vi "Open.vi"(8 "error in (no error)":errorcluster, 11 "Theory in":refnum<class "Theory.lvclass">) -> (0 "error out":errorcluster, 3 "Theory out":refnum<class "Theory.lvclass">)   [LabVIEW 2017, in "Theory.lvclass"]
doc: "Opens the test."
uses:
  Theory.lvclass
  Theory.lvclass/Theory.ctl
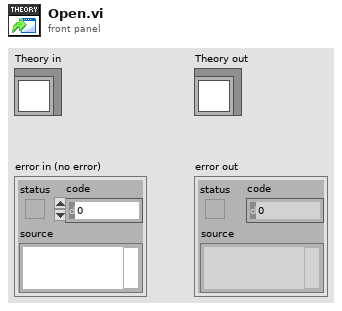
[diagram p1: front panel]
types:
  T1 = enum32{"Invalid", "Standard", "Closed", "Hidden", "Minimized", "Maximized"}
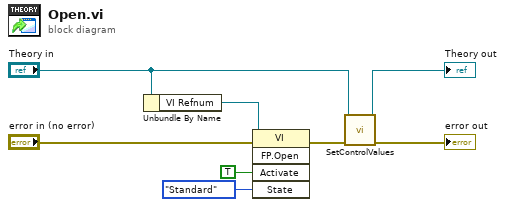
[diagram p0: block diagram]
diagram:
  n1 = Unbundle By Name("Theory in") -> ("VI Refnum"=w8:refnum<vi>)
  n2 = invoke class="VI" method="FP.Open"(reference=w8, error in="error in (no error)", "Activate"=TRUE ("Activate?"), "State"=T1."Standard") -> (error out=w4:errorcluster)  [unwired: 1 in, 4 out]
  n3 = call "SetControlValues.vi"("error in (no error)"=w4, "Theory in"="Theory in") -> ("error out"=→"error out":errorcluster, "Theory out"=→"Theory out":refnum<class "Theory.lvclass">)  [unwired: 8 in]
